vi "Shutdown.vi"(8 "error in (no error)":errorcluster, 11 "device data model in":refnum<class "ELAN Data Model.lvclass">) -> (0 "error out":errorcluster)   [LabVIEW 2021, in "ELAN Data Model.lvclass"]
doc: "This VI is responsible for deleting the device data model."
uses:
  ELAN Data Model.lvclass
  ELAN Data Model.lvclass/ELAN Data Model.ctl
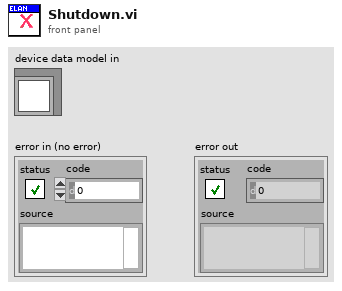
[diagram p1: front panel]
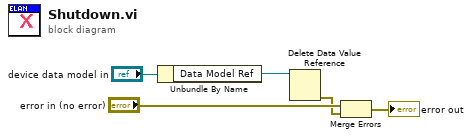
[diagram p0: block diagram]
diagram:
  n1 = Unbundle By Name("device data model in") -> ("Data Model Ref"=w4:refnum<data-value>)
  n2 = Delete Data Value Reference(data value reference=w4) -> (error out=w1:errorcluster)  [unwired: 1 in, 1 out]
  n3 = Merge Errors("error in (no error)", w1) -> (→"error out":errorcluster)
